vi "ExSubNframeCol_new_recovery.vi"(8 "error in (no error)":errorcluster, 9 "image handles":u32[](array[numeric]), 10 "Number of Images":u32=1 min=1 step=1, 11 "Handle Cluster 2":T1) -> (0 "error out":errorcluster, 1 "data handles":u32[](array[numeric]), 2 "x/y":dbl, 3 "Handle Cluster":T1, 4 "x > y?":bool, 5 "Frame Rate":dbl=1001.0010010010011, 6 "image #":i32)   [LabVIEW 2015]
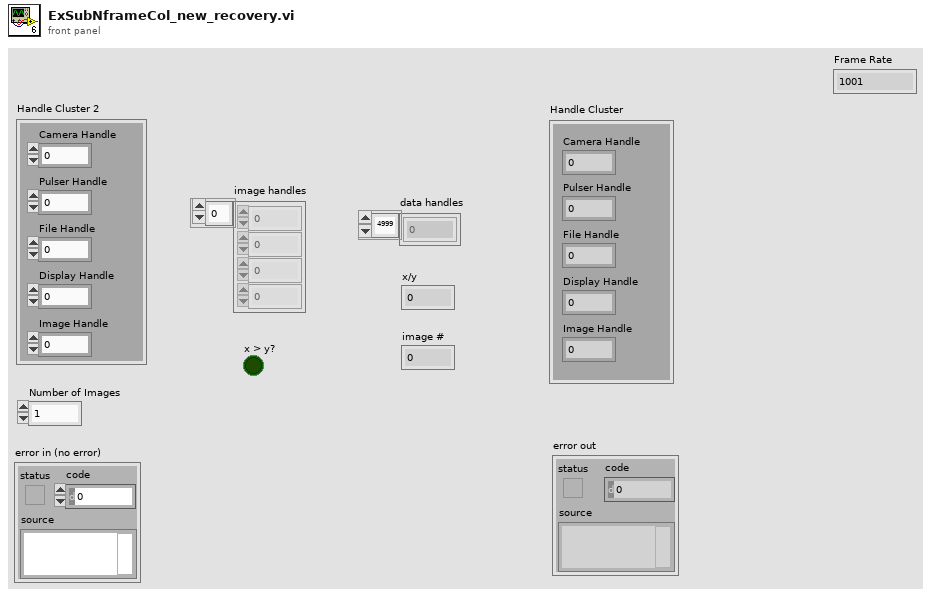
[diagram p1: front panel]
types:
  T1 = cluster{"Camera Handle":u32, "Pulser Handle":u32, "File Handle":u32, "Display Handle":u32, "Image Handle":u32}
  T2 = cluster{"Camera Handle":u32, "Pulser Handle":u32, "File Handle":u32, "Display Handle":u32, "Image/Data Handle":u32}
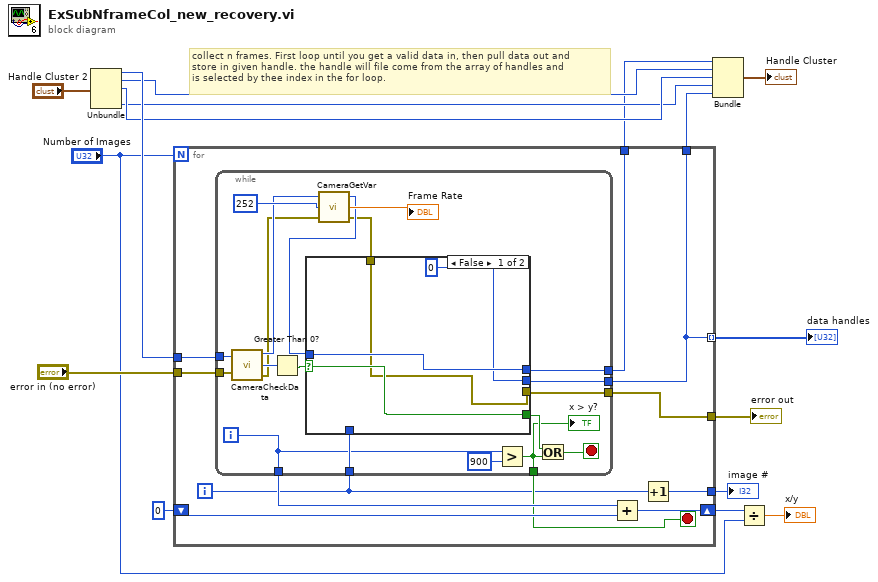
[diagram p0: block diagram]
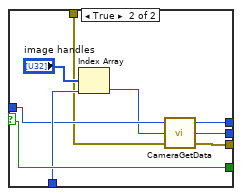
[diagram p2: hidden frame]
diagram:
  # "collect n frames. First loop until you get a valid data in, then pull data out and \nstore in given handle. the handle will file come from the array of handles and\nis selected by thee index in the for loop."
  n1 = Unbundle("Handle Cluster 2") -> ("Camera Handle"=w16:u32, "Pulser Handle"=w13:u32, "File Handle"=w12:u32, "Display Handle"=w11:u32)  [unwired: 1 out]
  n2 = for {
    N: "Number of Images" -> [_]
    tunnel: w16 -> [w27]
    tunnel: "error in (no error)" -> [w26]
    tunnel: [w25] -> w14
    tunnel: [w24] -> w8
    tunnel: [w23] -> w10
    tunnel: [w23] -> w9 mode=indexing
    shift-right: [w22] -> w4
    shift-left: 0 -> [w20]
    tunnel: [w17] -> w1
    i -> [w18]
    stop <- w19 stop-if-true
    n3 = while {
      tunnel: w26 -> [w40]
      tunnel: w27 -> [w41]
      tunnel: [w46] -> w25
      tunnel: w18 -> [w45]
      tunnel: [w44] -> w24
      tunnel: [w43] -> w23
      tunnel: [w34] -> w21
      tunnel: [w35] -> w19
      i -> [w34]
      stop <- w37 stop-if-true
      n4 = call <userlib>:"CameraCheckData.vi"("Camera Handle"=w41, "error in"=w40) -> ("Camera Handle"=w31:u32, "Number Of Frames Available"=w39:i32, "error out"=w29:errorcluster)
      n5 = Greater Than 0?(x=w39) -> (x > 0?=w42:bool)
      n6 = call <userlib>:"CameraGetVar.vi"("error in"=w29, "Parameter ID"=252, "Camera Handle"=w31) -> ("error out"=w28:errorcluster, "Value"=→"Frame Rate":dbl, "Camera Handle"=w30:u32)
      n7 = case shown="False" w42 {
        selector: w42 -> [w50 w59]
        tunnel: w30 -> [w49 w56]
        tunnel: [w50 w59] -> w38
        tunnel: [w47 w52] -> w46
        tunnel: w45 -> [_ w58]
        tunnel: [w49 w54] -> w44
        tunnel: [0 w53] -> w43
        tunnel: w28 -> [w47 w51]
        frame False {
        }
        frame True {
          n8 = Index Array(array="image handles", index=w58) -> (element=w55:u32)
          n9 = call <userlib>:"CameraGetData.vi"("error in"=w51, "Image/Data Handle"=w55, "Camera Handle"=w56) -> ("error out"=w52:errorcluster, "Image/Data Handle"=w53:u32, "Camera Handle"=w54:u32)
        }
      }
      n10 = Greater?(x=w34, y=900) -> (0:w35:bool)
      "x > y?" <- w35
      n11 = Or(x=w38, y=w35) -> (x .or. y?=w37:bool)
    }
    n12 = Add(x=w21, y=w20) -> (x+y=w22:i32)
    n13 = Increment(x=w18) -> (x+1=w17:i32)
  }
  "error out" <- w14
  "data handles" <- w9
  "image #" <- w1
  n14 = Bundle("Camera Handle"=w8, "Pulser Handle"=w13, "File Handle"=w12, "Display Handle"=w11, "Image/Data Handle"=w10) -> (→"Handle Cluster":T2)  [unwired: 1 in]
  n15 = Divide(x=w4, y="Number of Images") -> (x/y=→"x/y":dbl)
